vi "Conn Get Properties.vi"(4 "error in (no error)":errorcluster, 7 "connection reference":T2) -> (0 "error out":errorcluster, 1 "connection properties":T1, 3 "connection reference out":T2)   [LabVIEW 2012, in "NI_Database_API_64.lvlib"]
doc: "Gets properties of the object as determined by the inputs. This VI works for connections, commands, recordsets, columns, and parameters. Wire data to the reference input to determine the polymorphic instance to use or manually select the instance."
uses:
  NI_Database_API_64.lvlib
  Conn ObjectReference.ctl
  Conn Properties.ctl
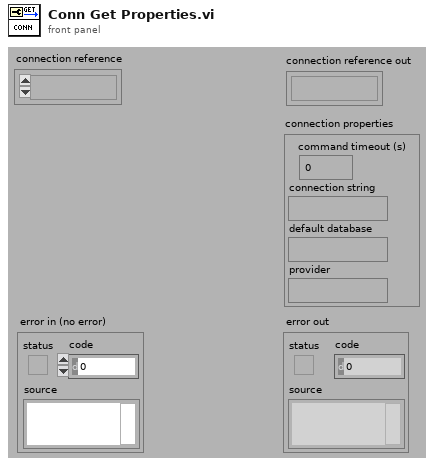
[diagram p1: front panel]
types:
  T1 = typedef "NI_Database_API_64.lvlib/Conn Properties.ctl" = cluster{"command timeout (s)":i32, "connection string":string, "default database":string, "provider":string}
  T2 = typedef "NI_Database_API_64.lvlib/Conn ObjectReference.ctl" = refnum<k1>
  T3 = typedef "NI_Database_API_64.lvlib/Conn DataMembers.ctl" = cluster{"ADODB._Connection":refnum<k7>, "recordset objects":i32, "command objects":i32}
  T4 = cluster{"CommandTimeout":i32, "ConnectionString":string, "DefaultDatabase":string, "Provider":string}
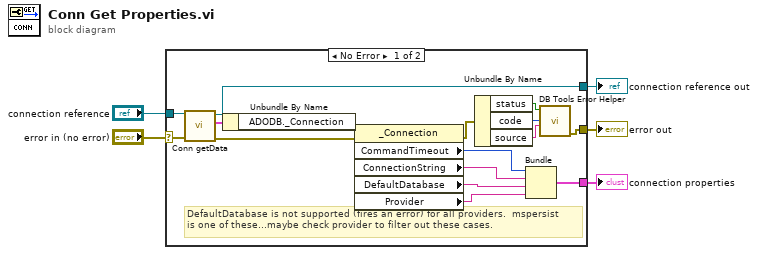
[diagram p0: block diagram]
diagram:
  n1 = case shown="No Error" "error in (no error)" {
    selector: "error in (no error)" -> [w6 w23]
    tunnel: "connection reference" -> [w21 w22]
    tunnel: [w16 _] -> w4
    tunnel: [w12 w22] -> w3
    tunnel: [w7 w23] -> w2
    frame No Error {
      # "DefaultDatabase is not supported (fires an error) for all providers.  mspersist\nis one of these...maybe check provider to filter out these cases."
      n2 = call "Conn getData.vi"("error in (no error)"=w6, "connection reference"=w21) -> ("error out"=w14:errorcluster, "data"=w15:T3, "connection reference out"=w12:T2)  [unwired: 3 out]
      n3 = Unbundle By Name(w15) -> ("ADODB._Connection"=w13:refnum<k7>)
      n4 = property class="_Connection"(reference=w13, error in=w14) -> (error out=w8:errorcluster, "CommandTimeout"=w20:i32, "ConnectionString"=w19:string, "DefaultDatabase"=w18:string, "Provider"=w17:string)  [unwired: 1 out]
      n5 = Unbundle By Name(w8) -> ("status"=w10:bool, "code"=w9:i32, "source"=w11:string)
      n6 = Bundle("CommandTimeout"=w20, "ConnectionString"=w19, "DefaultDatabase"=w18, "Provider"=w17) -> (w16:T4)  [unwired: 1 out]
      n7 = call "DB Tools Error Helper.vi"("source"=w11, "code"=w9, "status"=w10) -> ("error out"=w7:errorcluster)  [unwired: 1 in, 7 out]
    }
    frame Error {
    }
  }
  "connection reference out" <- w3
  "error out" <- w2
  "connection properties" <- w4
